vi "backup_data_on_network.vi"(7 "Application Directory":string, 11 "Filepath in":path) -> (3 "Filepath out":path)   [LabVIEW 2016]
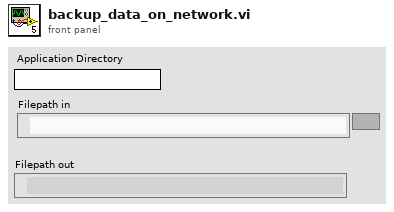
[diagram p1: front panel]
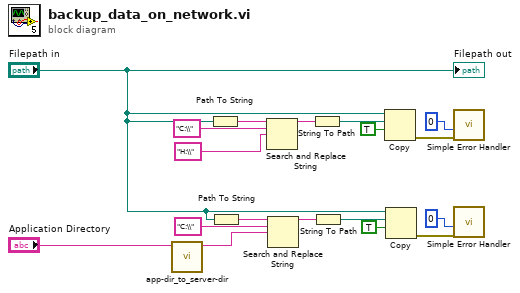
[diagram p0: block diagram]
diagram:
  n1 = call "app-dir_to_server-dir.vi"("Application Directory"="Application Directory") -> ("Group Server Directory"=w2:string)  [unwired: 10 in]
  n2 = Path To String(path="Filepath in") -> (string=w12:string)
  n3 = Path To String(path="Filepath in") -> (string=w7:string)
  n4 = Search and Replace String(input string=w12, search string="C:\\", replace string="H:\\") -> (result string=w14:string)  [unwired: 5 in, 3 out]
  n5 = Search and Replace String(input string=w7, search string="C:\\", replace string=w2) -> (result string=w9:string)  [unwired: 5 in, 3 out]
  n6 = String To Path(string=w14) -> (path=w13:path)
  n7 = String To Path(string=w9) -> (path=w8:path)
  n8 = Copy(9:TRUE ("overwrite (F)"), 10:w13, 11:"Filepath in") -> (0:w16:errorcluster)  [unwired: 2 in, 2 out]
  n9 = Copy(9:TRUE ("overwrite (F)"), 10:w8, 11:"Filepath in") -> (0:w18:errorcluster)  [unwired: 2 in, 2 out]
  n10 = call <vilib>:"Simple Error Handler.vi"("type of dialog (OK msg:1)"=0, "error in (no error)"=w16) -> ()  [unwired: 3 in, 5 out]
  n11 = call <vilib>:"Simple Error Handler.vi"("type of dialog (OK msg:1)"=0, "error in (no error)"=w18) -> ()  [unwired: 3 in, 5 out]
  "Filepath out" <- "Filepath in"
